vi "DCA Convert 1.8 to 1.9.vi"(0 "DCA 1.8 Test Parameters":T2={"Tag"="", "Use Instrument"=FALSE, "Quick Mode"=FALSE, "Topology"=enum."Pi", "Zo"=50.0, "Range"=0, "Resolution"=0, "Blank Screen"=FALSE, "Limits"=[], "Datasheets"={"Datasheets to Generate"=[], "Print Datasheets"=TRUE}, "Lock Topology"=FALSE, "Normalize"=TRUE, "ATTN Calc"=enum."Power"} {"Resolution" items=["Auto", "4 1/2", "5 1/2", "6 1/2"]; "Range" items=["Auto", "Min", "Max", "100", "1,000", "10,000", "100,000", "1,000,000", "10,000,000", "100,000,000"]; "Limits"."Run" min=1 step=1}) -> (1 "QuickMode":i8, 2 "DCA 1.9 Test Parameters":T1={"Stimulus"={"Use Instrument"=FALSE, "Normalize"=FALSE, "Blank Screen"=FALSE, "Measurement Type"=enum."Diode", "Range"=enum."Auto", "Resolution"=enum."Auto"}, "Measurement"={"Topology"=enum."PI-Network", "Lock Topology"=FALSE, "ATTN Calc"=enum."Power", "Zo"=50.0}, "Limits"=[], "Datasheets"=[]})   [LabVIEW 2011]
uses:
  TypeDefs/DCA Test Parameters v1.8.ctl
  TypeDefs/DCA Test Parameters v1.9.ctl
  TypeDefs/DCA Topology.ctl
panel:
  # "="
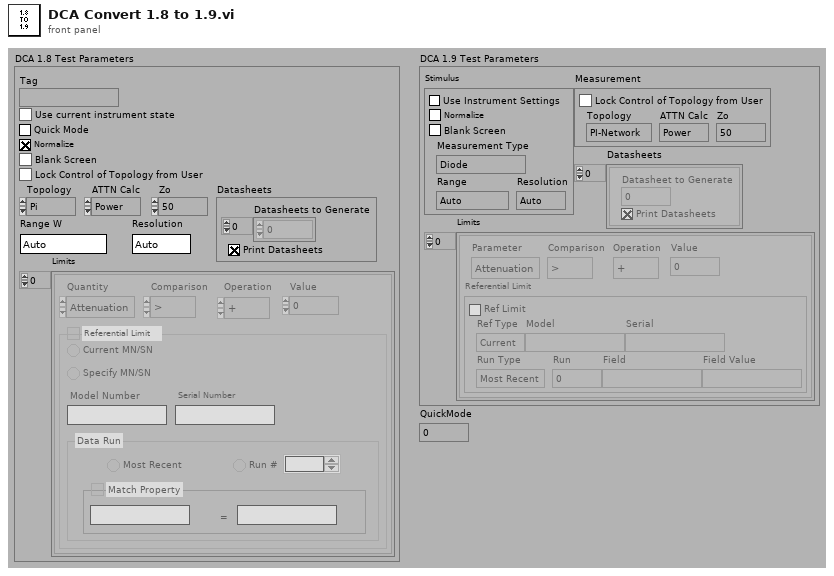
[diagram p1: front panel]
types:
  T1 = typedef "DCA Test Parameters v1.9.ctl" = cluster{"Stimulus":cluster{"Use Instrument":bool, "Normalize":bool, "Blank Screen":bool, "Measurement Type":enum16{"Voltage DC", "Voltage DC Ratio", "Voltage AC", "Current DC", "Current AC", "Resistance", "Fresistance", "Frequency", "Period", "Continuity", "Diode"}, "Range":enum16{"Auto", "Minimum", "Maximum", "100", "1,000", "10,000", "100,000", "1,000,000", "10,000,000", "100,000,000"}, "Resolution":enum16{"Auto", "4 1/2", "5 1/2", "6 1/2"}}, "Measurement":cluster{"Topology":enum32{"PI-Network", "T-Network"}, "Lock Topology":bool, "ATTN Calc":enum32{"Power", "Voltage"}, "Zo":dbl}, "Limits":cluster{"Parameter":enum16{"Attenuation", "Zin", "Zout", "R1", "R2", "R3", "Rab", "Rac", "Rbc"}, "Comparison":enum16{">", ">=", "<", "<="}, "Operation":enum16{"+", "-"}, "Value":dbl, "Referential Limit":cluster{"Ref Limit":bool, "Ref Type":enum16{"Current", "Specify"}, "Model":string, "Serial":string, "Run Type":enum16{"Most Recent", "Run #", "Match Field"}, "Run":i32, "Field":string, "Field Value":string}}[], "Datasheets":cluster{"Datasheet to Generate":i32, "Print Datasheets":bool}[]}
  T2 = typedef "DCA Test Parameters v1.8.ctl" = cluster{"Tag":string, "Use Instrument":bool, "Quick Mode":bool, "Topology":enum32{"Pi", "T"}, "Zo":dbl, "Range":u16, "Resolution":u16, "Blank Screen":bool, "Limits":cluster{"Quantity":enum16{"Attenuation", "Zin", "Zout", "R1", "R2", "R3", "Rab", "Rac", "Rbc"}, "Comparison":enum16{">", ">=", "<", "<=", "+", "-"}, "Operation":enum16{"+", "-"}, "Value":dbl, "Ref Limit":bool, "Ref Type":enum32{"Current", "Specify"}, "Model":string, "Serial":string, "Run Type":enum32{"Most Recent", "Run #"}, "Run":i32, "Match Property":bool, "Property":string, "Property Value":string}[], "Datasheets":cluster{"Datasheets to Generate":i32[], "Print Datasheets":bool}, "Lock Topology":bool, "Normalize":bool, "ATTN Calc":enum32{"Power", "Voltage"}}
  T3 = typedef "DCA Topology.ctl" = enum32{"PI-Network", "T-Network"}
  T4 = cluster{"Quantity":enum16{"Attenuation", "Zin", "Zout", "R1", "R2", "R3", "Rab", "Rac", "Rbc"}, "Comparison":enum16{">", ">=", "<", "<=", "+", "-"}, "Operation":enum16{"+", "-"}, "Value":dbl, "Ref Limit":bool, "Ref Type":enum32{"Current", "Specify"}, "Model":string, "Serial":string, "Run Type":enum32{"Most Recent", "Run #"}, "Run":i32, "Match Property":bool, "Property":string, "Property Value":string}[]
  T5 = cluster{"Parameter":enum16{"Attenuation", "Zin", "Zout", "R1", "R2", "R3", "Rab", "Rac", "Rbc"}, "Comparison":enum16{">", ">=", "<", "<="}, "Operation":enum16{"+", "-"}, "Value":dbl, "Referential Limit":cluster{"Ref Limit":bool, "Ref Type":enum16{"Current", "Specify"}, "Model":string, "Serial":string, "Run Type":enum16{"Most Recent", "Run #", "Match Field"}, "Run":i32, "Field":string, "Field Value":string}}[]
  T6 = cluster{"Datasheet to Generate":i32, "Print Datasheets":bool}[]
  T7 = cluster{"Datasheet to Generate":i32, "Print Datasheets":bool}
  T8 = cluster{"Parameter":enum16{"Attenuation", "Zin", "Zout", "R1", "R2", "R3", "Rab", "Rac", "Rbc"}, "Comparison":enum16{">", ">=", "<", "<="}, "Operation":enum16{"+", "-"}, "Value":dbl, "Referential Limit":cluster{"Ref Limit":bool, "Ref Type":enum16{"Current", "Specify"}, "Model":string, "Serial":string, "Run Type":enum16{"Most Recent", "Run #", "Match Field"}, "Run":i32, "Field":string, "Field Value":string}}
  T9 = enum16{"Attenuation", "Zin", "Zout", "R1", "R2", "R3", "Rab", "Rac", "Rbc"}
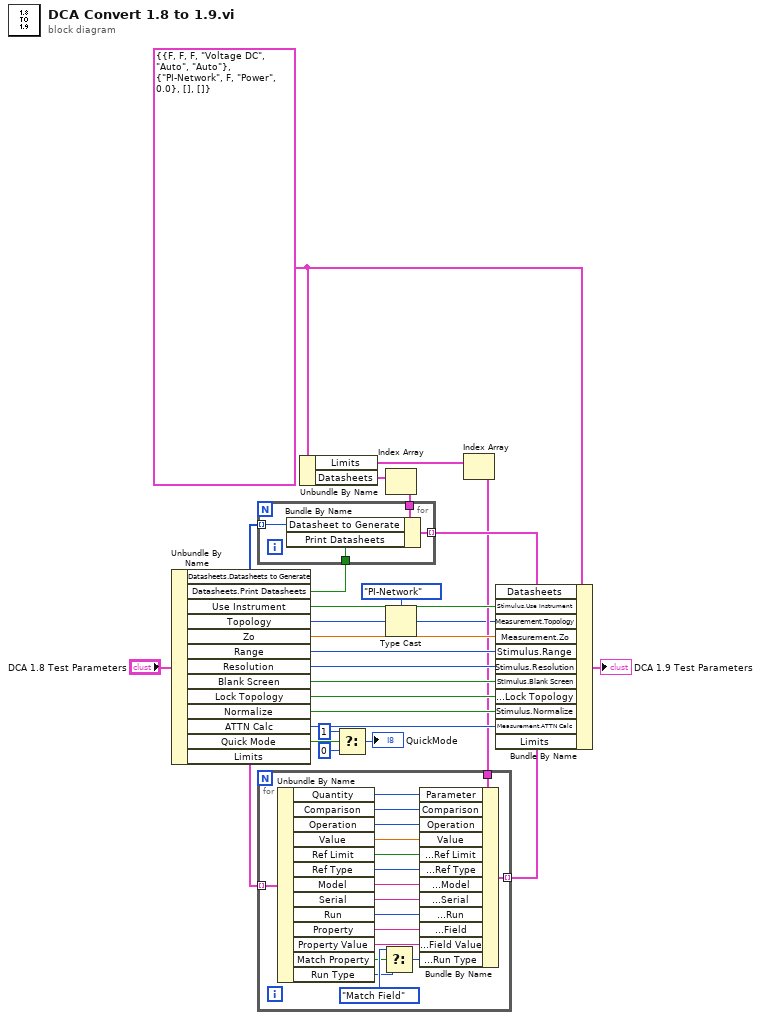
[diagram p0: block diagram]
diagram:
  w17 = T1 {"Stimulus"={"Use Instrument"=FALSE, "Normalize"=FALSE, "Blank Screen"=FALSE, "Measurement Type"=enum."Voltage DC", "Range"=enum."Auto", "Resolution"=enum."Auto"}, "Measurement"={"Topology"=enum."PI-Network", "Lock Topology"=FALSE, "ATTN Calc"=enum."Power", "Zo"=0.0}, "Limits"=[], "Datasheets"=[]} ("DCA 1.9 Test Parameters")
  n1 = Unbundle By Name("DCA 1.8 Test Parameters") -> ("Datasheets.Datasheets to Generate"=w13:i32[], "Datasheets.Print Datasheets"=w12:bool, "Use Instrument"=w25:bool, "Topology"=w7:enum32{"Pi", "T"}, "Zo"=w24:dbl, "Range"=w23:u16, "Resolution"=w22:u16, "Blank Screen"=w21:bool, "Lock Topology"=w20:bool, "Normalize"=w19:bool, "ATTN Calc"=w18:enum32{"Power", "Voltage"}, "Quick Mode"=w1:bool, "Limits"=w11:T4)
  n2 = Unbundle By Name(w17) -> ("Limits"=w10:T5, "Datasheets"=w16:T6)
  n3 = Select(t=i8 1 ("QuickMode"), s=w1, f=i8 0 ("QuickMode")) -> (s? t:f=→"QuickMode":i8)
  n4 = Index Array(array=w16) -> (element=w15:T7)  [unwired: 1 in]
  n5 = for {
    tunnel: w15 -> [w31]
    tunnel: [w30] -> w14 mode=indexing
    tunnel: w13 -> [w29] mode=indexing
    tunnel: w12 -> [w28]
    n6 = Bundle By Name(cluster=w31, "Datasheet to Generate"=w29, "Print Datasheets"=w28) -> (w30:T7)
  }
  n7 = Type Cast(type=DCA_Topology."PI-Network" ("Measurement.Topology"), x=w7) -> (*(type *) &x=w5:T3)
  n8 = Index Array(array=w10) -> (element=w9:T8)  [unwired: 1 in]
  n9 = for {
    tunnel: w11 -> [w49] mode=indexing
    tunnel: w9 -> [w48]
    tunnel: [w33] -> w8 mode=indexing
    n10 = Unbundle By Name(w49) -> ("Quantity"=w47:T9, "Comparison"=w46:enum16{">", ">=", "<", "<=", "+", "-"}, "Operation"=w45:enum16{"+", "-"}, "Value"=w44:dbl, "Ref Limit"=w43:bool, "Ref Type"=w32:enum32{"Current", "Specify"}, "Model"=w42:string, "Serial"=w41:string, "Run"=w40:i32, "Property"=w39:string, "Property Value"=w38:string, "Match Property"=w36:bool, "Run Type"=w35:enum32{"Most Recent", "Run #"})
    n11 = Select(t=enum32{"Most Recent", "Run #", "Match Field"}."Match Field" ("Run Type"), s=w36, f=w35) -> (s? t:f=w34:enum32{"Most Recent", "Run #", "Match Field"})
    n12 = Bundle By Name(cluster=w48, "Parameter"=w47, "Comparison"=w46, "Operation"=w45, "Value"=w44, "Referential Limit.Ref Limit"=w43, "Referential Limit.Ref Type"=w32, "Referential Limit.Model"=w42, "Referential Limit.Serial"=w41, "Referential Limit.Run"=w40, "Referential Limit.Field"=w39, "Referential Limit.Field Value"=w38, "Referential Limit.Run Type"=w34) -> (w33:T8)
  }
  n13 = Bundle By Name(cluster=w17, "Datasheets"=w14, "Stimulus.Use Instrument"=w25, "Measurement.Topology"=w5, "Measurement.Zo"=w24, "Stimulus.Range"=w23, "Stimulus.Resolution"=w22, "Stimulus.Blank Screen"=w21, "Measurement.Lock Topology"=w20, "Stimulus.Normalize"=w19, "Measurement.ATTN Calc"=w18, "Limits"=w8) -> (→"DCA 1.9 Test Parameters":T1)
